vi "Auto-Place.vi"   [LabVIEW 2018]
uses:
  Implementation/Drive Operations.ctl
  Framework/Robot Global Data.vi
types:
  T1 = typedef "Command Status Info.ctl" = cluster{"Name":string, "Status":T2, "notifier out":T3}
  T2 = typedef "Completion Status.ctl" = enum16{"Successful", "Aborted", "Incomplete"}
  T3 = typedef "Completion Notifier.ctl" = refnum<notifier>
  T4 = cluster{"Reverse (T) / Normal (F)":bool, "Power Scaling (1=Normal) ":dbl, "Deadband Value":dbl}
  T5 = typedef "Drive Operations.ctl" = enum16{"Reserve", "Read Current", "Immediate", "J-Turn", "Play Back From Log", "Auto-Align"}
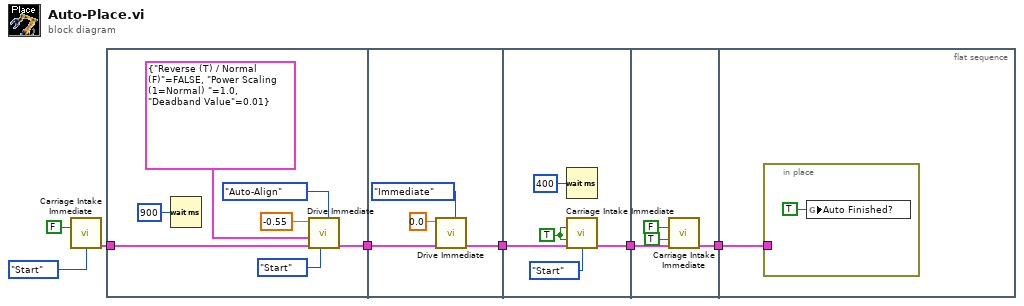
[diagram p0: block diagram]
diagram:
  n1 = call "Carriage Intake Immediate.vi"("Extend"=FALSE, "Synchronication"=enum16{"Start", "Wait"}."Start") -> ("Command Info Out"=w7:T1)  [unwired: 13 in]
  n2 = flat-sequence {
    tunnel: w7 -> [w11]
    tunnel: [w9] -> w5
    tunnel: w5 -> [w18]
    tunnel: [w17] -> w3
    tunnel: w3 -> [w23]
    tunnel: [w22] -> w2
    tunnel: w2 -> [w27]
    tunnel: [w25] -> w1
    tunnel: w1 -> [w28]
    frame #0 {
      n3 = Wait (ms)(milliseconds to wait=u32 900) -> ()  [unwired: 1 out]
      n4 = call "Drive Immediate.vi"("Operation"=Drive_Operations."Auto-Align", "Synchronication"=enum16{"Start", "Wait"}."Start", "Command Info In"=w11, "Modifiers"=T4 {"Reverse (T) / Normal (F)"=FALSE, "Power Scaling (1=Normal) "=1.0, "Deadband Value"=0.01}, "Left Setpoint (Power)"=-0.55) -> ("Command Info Out"=w9:T1)  [unwired: 6 in]
    }
    frame #1 {
      n5 = call "Drive Immediate.vi"("Operation"=Drive_Operations."Immediate", "Command Info In"=w18, "Left Setpoint (Power)"=0.0) -> ("Command Info Out"=w17:T1)  [unwired: 8 in]
    }
    frame #2 {
      w19 = TRUE ("Extend")
      n6 = Wait (ms)(milliseconds to wait=u32 400) -> ()  [unwired: 1 out]
      n7 = call "Carriage Intake Immediate.vi"("Extend"=w19, "Close"=w19, "Command Info In"=w23, "Synchronication"=enum16{"Start", "Wait"}."Start") -> ("Command Info Out"=w22:T1)  [unwired: 11 in]
    }
    frame #3 {
      n8 = call "Carriage Intake Immediate.vi"("Extend"=FALSE, "Close"=TRUE, "Command Info In"=w27) -> ("Command Info Out"=w25:T1)  [unwired: 12 in]
    }
    frame #4 {
      n9 = in-place {
        in-place-border: w28 -> [_]
        n10 = global write "Robot Global Data.vi" "Auto Finished?"(TRUE ("Auto Finished?")) -> ()
      }
    }
  }
